vi "PH_gentec_Powermeter.set modified data.vi"(0 "i ref in":refnum<vi>, 2 "i attribute":T1 {"Current Sets"."Data Sampling Settings"."Time Stamp" items=["Off", "On"]; "Current Sets"."Data Sampling Settings"."Total Duration Unit" items=["Period", "Seconds", "Minutes", "Hours", "Days", "Weeks", "Continuous", "# of Points"]; "Current Sets"."Data Sampling Settings"."Total Duration" max=300 step=1; "Current Sets"."Data Sampling Settings"."Sample Period Unit" items=["Seconds", "Minutes", "Hours", "Days", "Weeks", "Pulses"]; "Current Sets"."Data Sampling Settings"."Sample Rate Unit" items=["per Second", "per Minute", "per Hour", "per Day", "% pulses"]; "Current Sets"."Data Sampling Settings"."Sample Rate" max=300 step=1; "Wanted Sets"."Data Sampling Settings"."Time Stamp" items=["Off", "On"]; "Wanted Sets"."Data Sampling Settings"."Total Duration Unit" items=["Period", "Seconds", "Minutes", "Hours", "Days", "Weeks", "Continuous", "# of Points"]; "Wanted Sets"."Data Sampling Settings"."Total Duration" max=300 step=1; "Wanted Sets"."Data Sampling Settings"."Sample Period Unit" items=["Seconds", "Minutes", "Hours", "Days", "Weeks", "Pulses"]; "Wanted Sets"."Data Sampling Settings"."Sample Rate Unit" items=["per Second", "per Minute", "per Hour", "per Day", "% pulses"]; "Wanted Sets"."Data Sampling Settings"."Sample Rate" max=300 step=1}, 5 "error in (no error)":errorcluster) -> (14 "i ref out":refnum<vi>, 19 "error out":errorcluster)   [LabVIEW 2014, in "PH_gentec_Powermeter.lvlib"]
doc: "Writes the data into the attribute of an object. Then, the attribute dara are unlocked using the \"release\" method. Prior to calling THIS method, the attribute data must have been locked using the methods \"lock\" or \"get data to modify\".\n\n\nLicense Agreement for this software:\n\nCopyright (C)\nGesellschaft für Schwerionenforschung, GSI\nPlanckstr. 1\n64291 Darmstadt\nGermany\n\nContact: D.Beck@gsi.de \n\nThis program is free software; you can redistribute it and/or modify it under the terms of the GNU General Public License as published by the Free Software Foundation; either version 2 of the license, or (at your option) any later version.\n\nThis program is distributed in the hope that it will be useful, but WITHOUT ANY WARRANTY; without even the implied warranty of MERCHANTABILITY or FITNESS FOR A PARTICULAR PURPOSE. See the GNU General License for more details (http://www.gnu.org).\n\nGesellschaft für Schwerionenforschung, GSI\nPlanckstr. 1, 64291 Darmstadt, Germany\nFor all questions and ideas contact: M.Richter@gsi.de, H.Brand@gsi.de or D.Beck@gsi.de.\nLast update: 17-JUN-2004"
uses:
  PH_gentec_Powermeter.lvlib
  PH_gentec_Powermeter.i attribute.ctl
  non_GPL/instr.lib/gentec-SOLO-PE/Driver/Type Defs/gentec-SOLO-PE.Statistics Data.ctl
  non_GPL/instr.lib/gentec-SOLO-PE/Driver/Type Defs/gentec-SOLO-PE.Configuration Values.ctl
  non_GPL/instr.lib/gentec-SOLO-PE/Driver/Type Defs/gentec-SOLO-PE.Scale.ctl
  non_GPL/instr.lib/gentec-SOLO-PE/Driver/Type Defs/gentec-SOLO-PE.Data Sampling Settings.ctl
  PH_gentec_Powermeter.Sets.ctl
  CSCore/CSObj/CSObj.lvlib
  non_GPL/instr.lib/gentec-SOLO-PE/gentec-SOLO-PE - Driver.lvlib
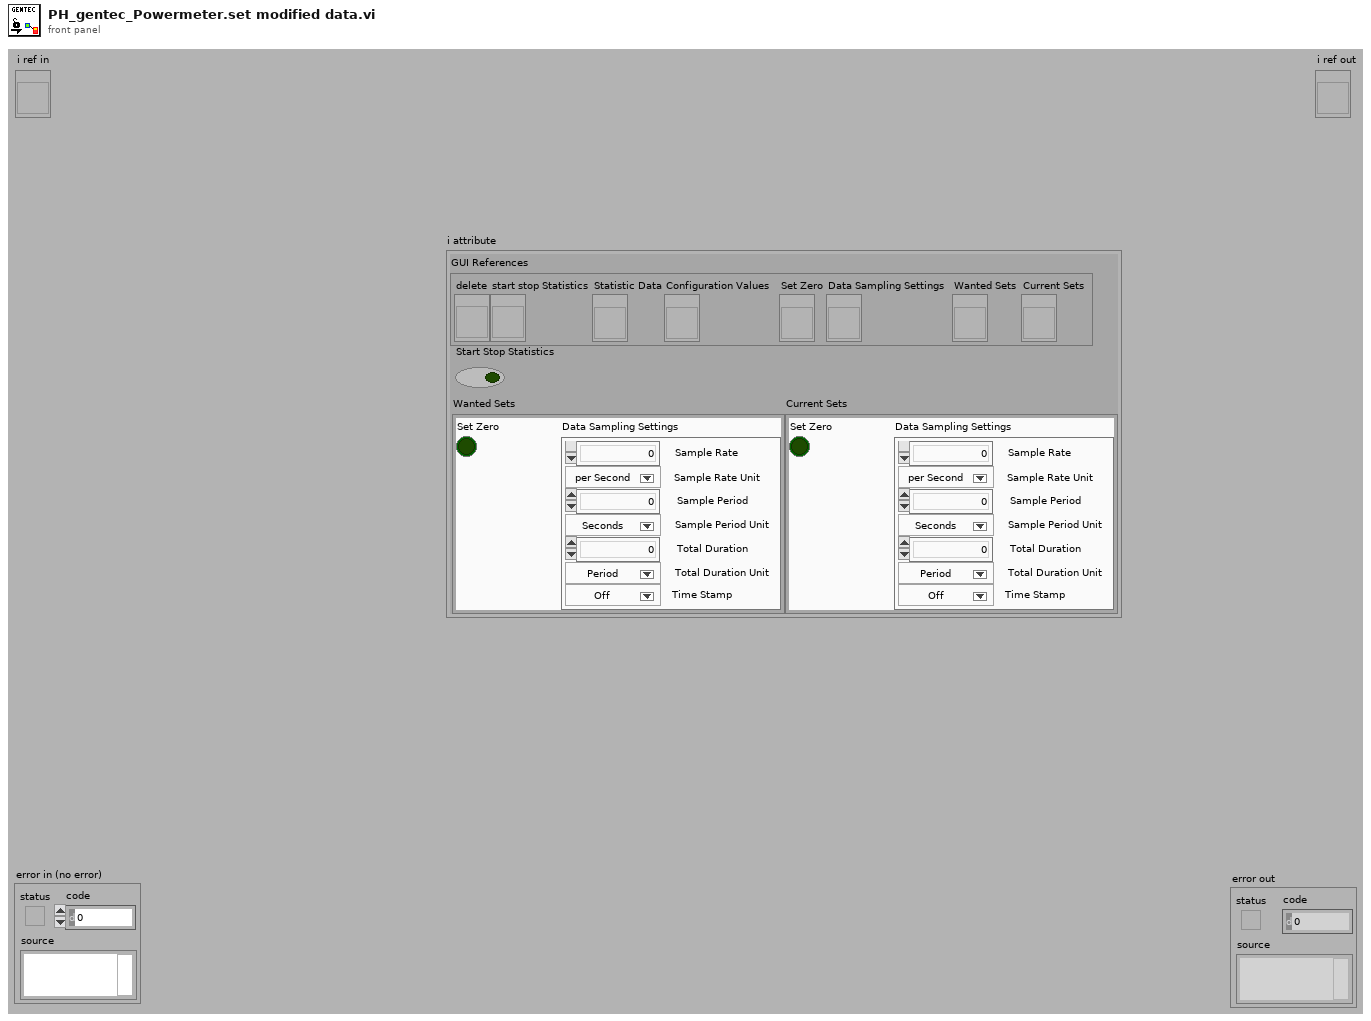
[diagram p1: front panel]
types:
  T1 = typedef "PH_gentec_Powermeter.lvlib/PH_gentec_Powermeter.i attribute.ctl" = cluster{"GUI References":cluster{"delete":refnum<vi>, "start stop Statistics":refnum<vi>, "Statistic Data":refnum<vi>, "Configuration Values":refnum<vi>, "Set Zero":refnum<vi>, "Data Sampling Settings":refnum<vi>, "Wanted Sets":refnum<vi>, "Current Sets":refnum<vi>}, "Start Stop Statistics":bool, "Wanted Sets":T2, "Current Sets":T2}
  T2 = typedef "PH_gentec_Powermeter.lvlib/PH_gentec_Powermeter.Sets.ctl" = cluster{"Data Sampling Settings":T3, "Set Zero":bool}
  T3 = typedef "gentec-SOLO-PE - Driver.lvlib/gentec-SOLO-PE.Data Sampling Settings.ctl" = cluster{"Sample Rate":u32, "Sample Rate Unit":u32, "Sample Period":u32, "Sample Period Unit":u32, "Total Duration":u32, "Total Duration Unit":u32, "Time Stamp":u32}
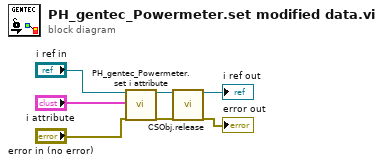
[diagram p0: block diagram]
diagram:
  n1 = call "PH_gentec_Powermeter.set i attribute.vi"("i ref in"="i ref in", "i attribute"="i attribute", "error in (no error)"="error in (no error)") -> ("i ref out"=w4:refnum<vi>, "error out"=w3:errorcluster)  [unwired: 15 in]
  n2 = call "CSObj.release.vi"("i ref in"=w4, "error in (no error)"=w3) -> ("i ref out"=→"i ref out":refnum<vi>, "error out"=→"error out":errorcluster)  [unwired: 16 in]
